vi "UI.StationUpdate.vi"(8 "error in (no error)":errorcluster, 11 "state variables":T1) -> (0 "error out":errorcluster)   [LabVIEW 2015, in "Stations.Overview.lvlib"]
uses:
  Stations.Overview.lvlib
  Types/Overview.StateVariables.ctl
  Types/Overview.Channels.ctl
  <vilib>/NI Veristand/Execution/Workspace/SystemStateEventRef.ctl
  <vilib>/NI Veristand/Execution/Workspace/Target State Info.ctl
  <vilib>/NI Veristand/Execution/Workspace/Target State.ctl
  <vilib>/NI Veristand/Execution/Workspace/WorkspaceAPI.ctl
  NationalInstruments.VeriStand.ClientAPI
  Execution GUI/Types/Execute.UserEventRefs.ctl
  <vilib>/NI Veristand/Execution/Workspace/SystemStateRegEventRef.ctl
  <vilib>/NI Veristand/Execution/WaveformStreaming/Waveform Data Watcher Event Data (DBL).ctl
  <vilib>/NI Veristand/Execution/WaveformStreaming/WaveformStreamSpecification.ctl
  <vilib>/NI Veristand/Execution/Workspace/NI VeriStand - Get Multiple Channel Values.vi
  <vilib>/NI Veristand/Execution/Workspace/NI_VS Workspace ExecutionAPI.lvlib
  Execution GUI/Station.Execution.lvlib
  <vilib>/NI Veristand/Execution/WaveformStreaming/NI_VS Waveform Streaming Interface.lvlib
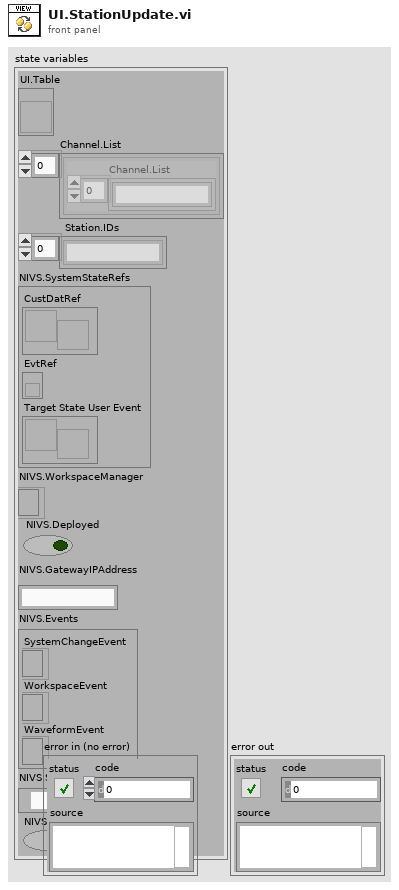
[diagram p1: front panel]
types:
  T1 = typedef "Stations.Overview.lvlib/Overview.StateVariables.ctl" = cluster{"UI.Table":refnum<vi>, "Channel.List":T2[], "Station.IDs":string[], "NIVS.SystemStateRefs":T3, "NIVS.WorkspaceManager":T4, "NIVS.Deployed":bool, "NIVS.GatewayIPAddress":string, "NIVS.Events":T5, "NIVS.SystemDefinitionFile":path, "NIVS.Open":bool}
  T2 = typedef "Stations.Overview.lvlib/Overview.Channels.ctl" = cluster{"Channel.List":string[]}
  T3 = typedef "NI_VS Workspace ExecutionAPI.lvlib/SystemStateEventRef.ctl" = cluster{"CustDatRef":refnum<user-event>, "EvtRef":refnum<k27>, "Target State User Event":refnum<user-event>}
  T4 = typedef "NI_VS Workspace ExecutionAPI.lvlib/WorkspaceAPI.ctl" = refnum<k24>
  T5 = typedef "Station.Execution.lvlib/Execute.UserEventRefs.ctl" = cluster{"SystemChangeEvent":T6, "WorkspaceEvent":refnum<event-registration>, "WaveformEvent":refnum<event-registration>}
  T6 = typedef "NI_VS Workspace ExecutionAPI.lvlib/SystemStateRegEventRef.ctl" = refnum<event-registration>
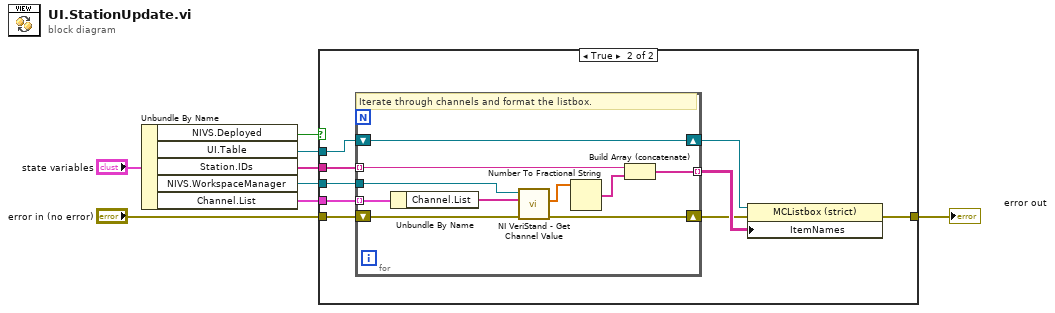
[diagram p0: block diagram]
diagram:
  n1 = Unbundle By Name("state variables") -> ("NIVS.Deployed"=w1:bool, "UI.Table"=w7:refnum<vi>, "Station.IDs"=w8:string[], "NIVS.WorkspaceManager"=w4:T4, "Channel.List"=w3:T2[])
  n2 = case shown="True" w1 {
    tunnel: w8 -> [_ w18]
    tunnel: w7 -> [_ w17]
    tunnel: "error in (no error)" -> [w9 w16]
    tunnel: w4 -> [_ w15]
    tunnel: w3 -> [_ w14]
    tunnel: [w9 w10] -> w2
    frame False {
    }
    frame True {
      n3 = for {
        shift-right: [w19] -> w11
        shift-left: w16 -> [w24]
        tunnel: w18 -> [w26] mode=indexing
        tunnel: [w28] -> w13 mode=indexing
        tunnel: w15 -> [w27]
        tunnel: w14 -> [w21] mode=indexing
        shift-right: [w25] -> w12
        shift-left: w17 -> [w25]
        # "Iterate through channels and format the listbox."
        n4 = Unbundle By Name(w21) -> ("Channel.List"=w20:string[])
        n5 = call-poly <vilib>:"NI VeriStand - Get Channel Value.vi"("error in (no error)"=w24, "Channels"=w20, "WorkspaceManager in"=w27) -> ("error out"=w19:errorcluster, "Values"=w23:dbl[])  [unwired: 6 in, 1 out]
        n6 = Number To Fractional String(number=w23) -> (F-format string=w22:string[])  [unwired: 3 in]
        n7 = Build Array (concatenate)(w26, w22) -> (w28:string[])
      }
      n8 = property class="MCListbox (strict)"(reference=w12, error in=w11, "ItemNames"=w13) -> (error out=w10:errorcluster)  [unwired: 1 out]
    }
  }
  "error out" <- w2
